vi "Baby Shark GUID Lookup.vi"() -> ()   [LabVIEW 2018, in "Baby Shark Custom Device.lvlib"]
doc: "Use this Global VI to access the GUIDs assigned to the page resources of the Custom Device."
uses:
  Baby Shark Custom Device.lvlib
panel:
  in  "Custom Device":string="3017f3fb-8eca-4813-a685-5e38ed020d92"
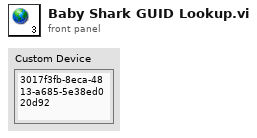
[diagram p1: front panel]
diagram:
